vi "parse_digital_io_state.vi"(4 "error in":errorcluster, 7 "msg in":string) -> (0 "error out":errorcluster, 2 "Digital IO State":cluster{"state":i8, "is input only":bool}, 3 "msg out":string)   [LabVIEW 2012]
uses:
  <userlib>/rosforlv/ROS/parsing/std_msgs/subs/parse_i8_scalar.vi
  <userlib>/rosforlv/ROS/parsing/std_msgs/subs/parse_bool_scalar.vi
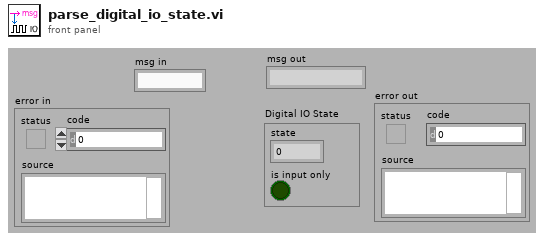
[diagram p1: front panel]
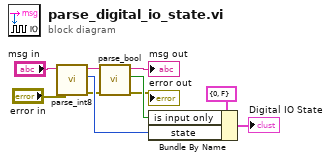
[diagram p0: block diagram]
diagram:
  n1 = call-poly <userlib>:"parse_int8.vi"("error in"="error in", "msg in"="msg in") -> ("error out"=w3:errorcluster, "number"=w4:i8, "msg out"=w9:string)  [unwired: 3 in]
  n2 = call-poly <userlib>:"parse_bool.vi"("error in"=w3, "msg in"=w9) -> ("error out"=→"error out":errorcluster, "bool"=w5:bool, "msg out"=→"msg out":string)  [unwired: 3 in]
  n3 = Bundle By Name(cluster=cluster{"state":i8, "is input only":bool} {"state"=0, "is input only"=FALSE} ("Digital IO State"), "is input only"=w5, "state"=w4) -> (→"Digital IO State":cluster{"state":i8, "is input only":bool})
